vi "set zone.vi"(11 "Cell.lvclass in":refnum<class "Cell.lvclass">) -> (3 "Cell.lvclass out":refnum<class "Cell.lvclass">)   [LabVIEW 2021, in "Cell.lvclass"]
uses:
  Cell.lvclass
  Cell.lvclass/Cell.ctl
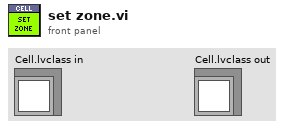
[diagram p1: front panel]
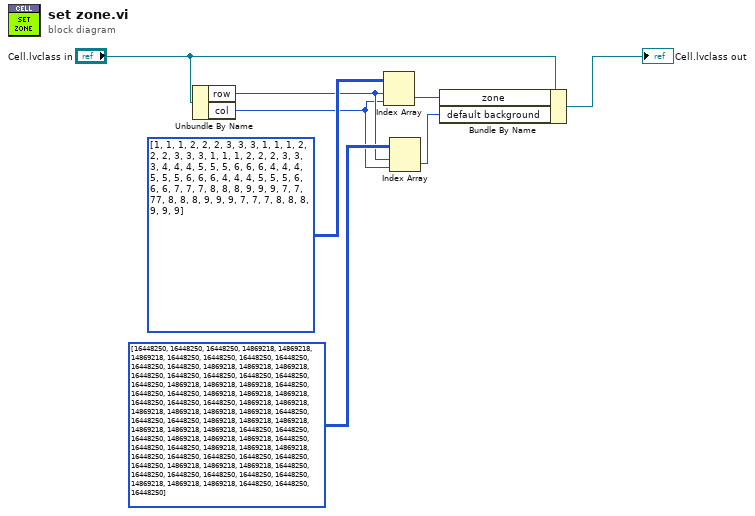
[diagram p0: block diagram]
diagram:
  n1 = Unbundle By Name("Cell.lvclass in") -> ("row"=w3:i32, "col"=w2:i32)
  n2 = Index Array(array=i32[][] [[1, 1, 1, 2, 2, 2, 3, 3, 3], [1, 1, 1, 2, 2, 2, 3, 3, 3], [1, 1, 1, 2, 2, 2, 3, 3, 3], [4, 4, 4, 5, 5, 5, 6, 6, 6], [4, 4, 4, 5, 5, 5, 6, 6, 6], [4, 4, 4, 5, 5, 5, 6, 6, 6], [7, 7, 7, 8, 8, 8, 9, 9, 9], [7, 7, 77, 8, 8, 8, 9, 9, 9], [7, 7, 7, 8, 8, 8, 9, 9, 9]], index (row)=w3, index (col)=w2) -> (element=w5:i32)
  n3 = Index Array(array=u32[][] [[16448250, 16448250, 16448250, 14869218, 14869218, 14869218, 16448250, 16448250, 16448250], [16448250, 16448250, 16448250, 14869218, 14869218, 14869218, 16448250, 16448250, 16448250], [16448250, 16448250, 16448250, 14869218, 14869218, 14869218, 16448250, 16448250, 16448250], [14869218, 14869218, 14869218, 16448250, 16448250, 16448250, 14869218, 14869218, 14869218], [14869218, 14869218, 14869218, 16448250, 16448250, 16448250, 14869218, 14869218, 14869218], [14869218, 14869218, 14869218, 16448250, 16448250, 16448250, 14869218, 14869218, 14869218], [16448250, 16448250, 16448250, 14869218, 14869218, 14869218, 16448250, 16448250, 16448250], [16448250, 16448250, 16448250, 14869218, 14869218, 14869218, 16448250, 16448250, 16448250], [16448250, 16448250, 16448250, 14869218, 14869218, 14869218, 16448250, 16448250, 16448250]], index (row)=w3, index (col)=w2) -> (element=w1:u32)
  n4 = Bundle By Name(cluster="Cell.lvclass in", "zone"=w5, "default background"=w1) -> (→"Cell.lvclass out":refnum<class "Cell.lvclass">)
